vi "PID Tuner UDP.vi"() -> ()   [LabVIEW 2017]
panel:
  in  "IP":string="10.1.95.2"
  out "Integral Accum":dbl
  in  "IZone":dbl
  in  "RampRate":dbl
  in  "Acceleration":dbl
  in  "Cruise Velocity":dbl
  in  "Reset Average":bool=TRUE
  out "Average Deviation":dbl
  out "Deviation Plot":dynamicdata(graph)=[{"t0"=timestamp(3600540520.2268195 s since 1904-01-01), "dt"=1.0, "Y"=[0.0]}, {"t0"=timestamp(3600540520.2268195 s since 1904-01-01), "dt"=1.0, "Y"=[0.0]}]
  out "Deviation":dbl
  in  "Setpoint":dbl
  in  "f":dbl
  in  "kD":dbl
  in  "kI":dbl
  in  "kP":dbl
  in  "port":u16=5807
  out "Name":string
  out "ActualValue":dbl
  out "DesiredValue":dbl
  out "Actual vs. Desired":dynamicdata(graph)=[{"t0"=timestamp(3600540520.2268195 s since 1904-01-01), "dt"=1.0, "Y"=[0.0]}, {"t0"=timestamp(3600540520.2268195 s since 1904-01-01), "dt"=1.0, "Y"=[0.0]}]
  # ".32"
  # ".00026"
  # "18"
  # ".076"
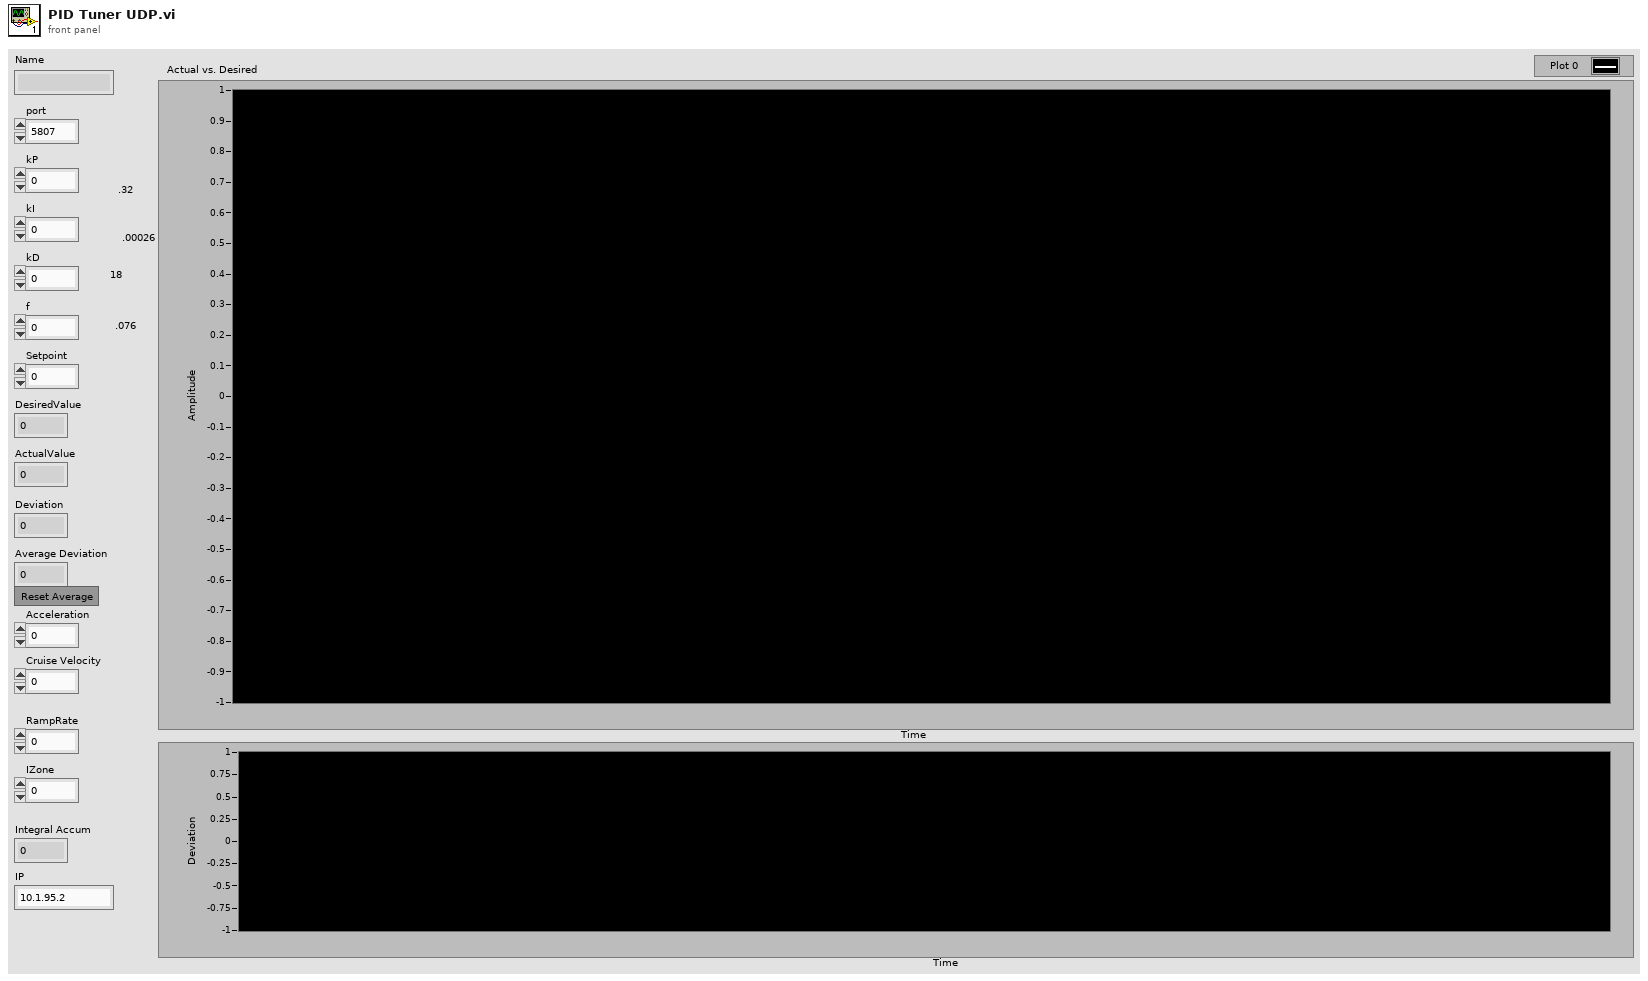
[diagram p1: front panel]
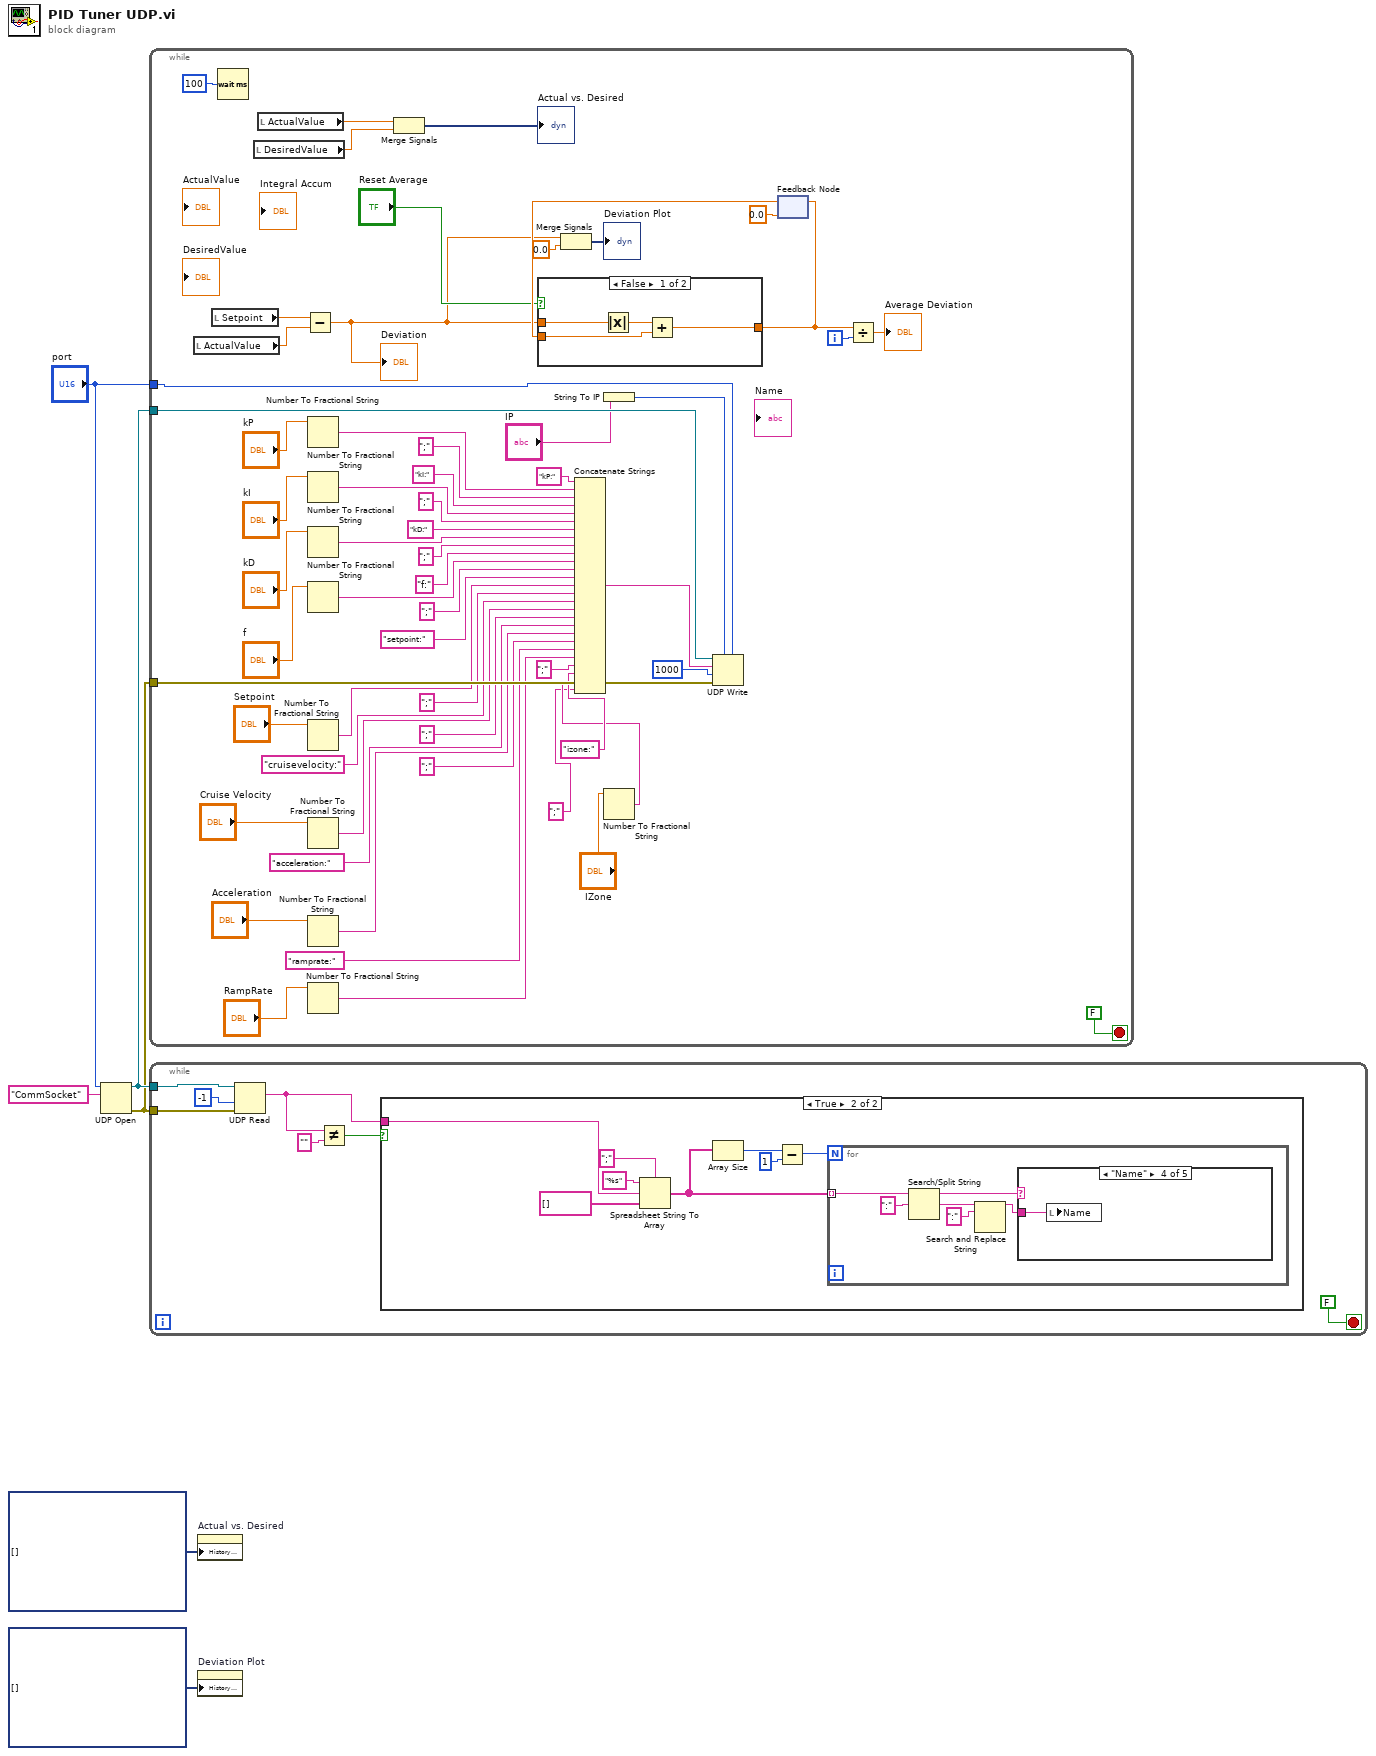
[diagram p0: block diagram]
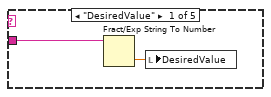
[diagram p3: hidden frame]
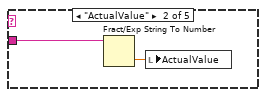
[diagram p4: hidden frame]
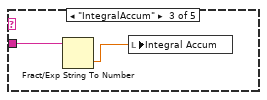
[diagram p5: hidden frame]
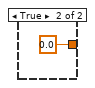
[diagram p7: hidden frame]
diagram:
  n1 = UDP Open(10:"CommSocket" ("service name"), 11:"port") -> (port=w4:refnum<k16>, 0:w3:errorcluster)  [unwired: 3 in, 1 out]
  n2 = while {
    tunnel: w4 -> [w62]
    tunnel: w3 -> [w61]
    tunnel: "port" -> [w59]
    i -> [w28]
    stop <- FALSE stop-if-true
    n3 = local read "ActualValue"() -> (w32:dbl)
    n4 = local read "Setpoint"() -> (w33:dbl)
    n5 = Wait (ms)(milliseconds to wait=u32 100) -> ()  [unwired: 1 out]
    n6 = local read "DesiredValue"() -> (w64:dbl)
    n7 = local read "ActualValue"() -> (w65:dbl)
    n8 = Subtract(x=w33, y=w32) -> (x-y=w25:dbl)
    "Deviation" <- w25
    n9 = Number To Fractional String(number="kP") -> (F-format string=w56:string)  [unwired: 3 in]
    n10 = Number To Fractional String(number="kI") -> (F-format string=w52:string)  [unwired: 3 in]
    n11 = Number To Fractional String(number="kD") -> (F-format string=w49:string)  [unwired: 3 in]
    n12 = Number To Fractional String(number="f") -> (F-format string=w46:string)  [unwired: 3 in]
    n13 = Number To Fractional String(number="Setpoint") -> (F-format string=w36:string)  [unwired: 3 in]
    n14 = Number To Fractional String(number="Cruise Velocity") -> (F-format string=w20:string)  [unwired: 3 in]
    n15 = Number To Fractional String(number="Acceleration") -> (F-format string=w16:string)  [unwired: 3 in]
    n16 = Number To Fractional String(number="RampRate") -> (F-format string=w12:string)  [unwired: 3 in]
    n17 = Merge Signals(w65, w64) -> (→"Actual vs. Desired":dynamicdata)
    n18 = Merge Signals(w25, 0.0) -> (→"Deviation Plot":dynamicdata)
    n19 = String To IP(1:"IP") -> (0:w60:u32)
    n20 = Number To Fractional String(number="IZone") -> (F-format string=w9:string)  [unwired: 3 in]
    n21 = Concatenate Strings("kP:", w56, ";", "kI:", w52, ";", "kD:", w49, ";", "f:", w46, ";", "setpoint:", w36, ";", "cruisevelocity:", w20, ";", "acceleration:", w16, ";", "ramprate:" ("string"), w12, ";", "izone:" ("string"), w9, ";") -> (w40:string)
    n22 = UDP Write(address=w60, port or service name=w59, connection ID=w62, data in=w40, 8:w61, 9:1000 ("timeout ms (25000)")) -> ()  [unwired: 2 out]
    n23 = feedback #1(0.0) -> (w31:dbl)
    n24 = case shown="False" "Reset Average" {
      tunnel: w25 -> [w69 _]
      tunnel: w31 -> [w68 _]
      tunnel: [w67 0.0] -> w29
      frame False {
        n25 = Absolute Value(x=w69) -> (abs(x)=w66:dbl)
        n26 = Add(x=w66, y=w68) -> (x+y=w67:dbl)
      }
      frame True {
      }
    }
    n27 = feedback-in #1(w29) -> ()
    n28 = Divide(x=w29, y=w28) -> (x/y=→"Average Deviation":dbl)
  }
  n29 = while {
    tunnel: w4 -> [w73]
    tunnel: w3 -> [w72]
    stop <- FALSE stop-if-true
    n30 = UDP Read(connection ID=w73, timeout ms (25000)=-1, 8:w72) -> (data out=w77:string)  [unwired: 1 in, 4 out]
    n31 = Not Equal?(x=w77, y="") -> (x != y?=w76:bool)
    n32 = case shown="True" w76 {
      tunnel: w77 -> [_ w85]
      frame False {
      }
      frame True {
        n33 = Spreadsheet String To Array(delimiter (Tab)=";" ("search string/char (-)"), format string="%s", spreadsheet string=w85, array type (2D Dbl)=string[] []) -> (array=w81:string[])
        n34 = Array Size(array=w81) -> (size(s)=w80:i32)
        n35 = Subtract(x=w80, y=1) -> (x-y=w78:i32)
        n36 = for {
          N: w78 -> [_]
          tunnel: w81 -> [w91] mode=indexing
          n37 = Search/Split String(string=w91, search string/char (-)=":") -> (substring before match=w89:string, match + rest of string=w88:string)  [unwired: 1 in, 1 out]
          n38 = Search and Replace String(input string=w88, search string=":" ("replace string (\"\")")) -> (result string=w86:string)  [unwired: 6 in, 3 out]
          n39 = case shown="\"Name\"" w89 {
            tunnel: w86 -> [w93 w95 w97 w98 _]
            frame "DesiredValue" {
              n40 = Fract/Exp String To Number(string=w93) -> (number=w92:dbl)  [unwired: 3 in, 1 out]
              n41 = local write "DesiredValue"(w92) -> ()
            }
            frame "ActualValue" {
              n42 = Fract/Exp String To Number(string=w95) -> (number=w94:dbl)  [unwired: 3 in, 1 out]
              n43 = local write "ActualValue"(w94) -> ()
            }
            frame "IntegralAccum" {
              n44 = Fract/Exp String To Number(string=w97) -> (number=w96:dbl)  [unwired: 3 in, 1 out]
              n45 = local write "Integral Accum"(w96) -> ()
            }
            frame "Name" {
              n46 = local write "Name"(w98) -> ()
            }
            frame "False", Default {
            }
          }
        }
      }
    }
  }
  n47 = property on="Actual vs. Desired" class="WFChart (strict)"("History Data"=dynamicdata[] []) -> ()  [unwired: 2 in, 2 out]
  n48 = property on="Deviation Plot" class="WFChart (strict)"("History Data"=dynamicdata[] []) -> ()  [unwired: 2 in, 2 out]
